vi "RT Microprocessor.vi"() -> ()   [LabVIEW 2014]
uses:
  <vilib>/FPGAPlugInAG/sbRIO-9636/niLvFpga_Open_sbRIO-9636.vi
  <vilib>/rvi/interface/common/dynamic/niFpgaDynamicAddResources.vi
  <vilib>/EmbeddedDisplay/Hitachi HD44780/Host/Public/Output (String).vi
  <vilib>/rvi/interface/nirviOpenFPGA/nirviOpenFPGA.xnode
  FPGA Bitfiles/Exercise1-OpenRu_FPGATarget_Exercise1Openand_49511F73.lvbitx
  <vilib>/EmbeddedDisplay/Hitachi HD44780/Host/HD44780 Host.lvlib
panel:
  in  "Direction":bool
  in  "Text":string="NI LabVIEW RIO Architecture"
  in  "stop":bool
  # "This VI writes the text you specify on the LCD device,\nand then shifts the text to the left or the right."
  # "Output Configuration"
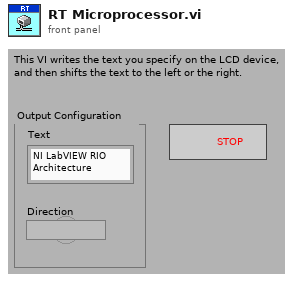
[diagram p1: front panel]
types:
  T1 = enum8{"5x8 & 2 lines", "5x10 & 1 line", "5x8 & 1 line"}
  T2 = enum8{"8x1", "8x2", "12x4", "16x1", "16x2", "16x4", "20x1", "20x2", "20x4", "24x1", "24x2", "40x2", "40x4"}
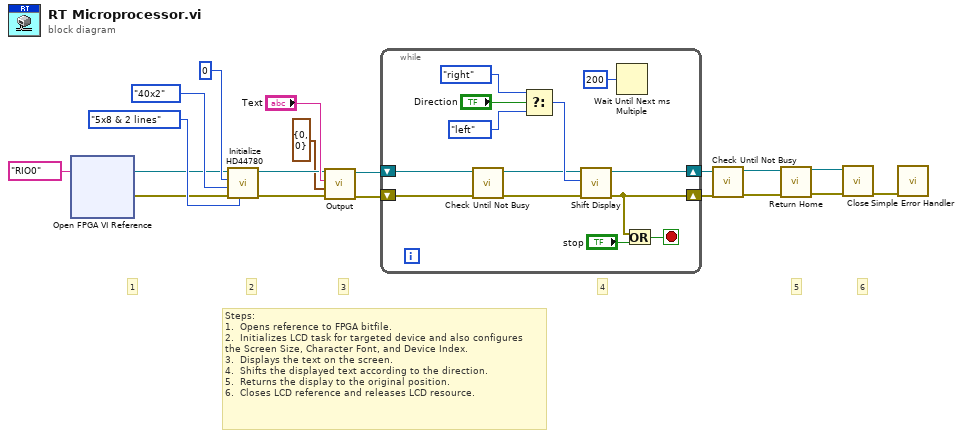
[diagram p0: block diagram]
diagram:
  # "6"
  # "5"
  # "4"
  # "3"
  # "2"
  # "1"
  # "Steps:  \n1.  Opens reference to FPGA bitfile.\n2.  Initializes LCD task for targeted device and also configures\nthe Screen Size, Character Font, and Device Index.\n3.  Displays the text on the screen.\n4.  Shifts the displayed text according to the direction.\n5.  Returns the display to the original position.\n6.  Closes LCD reference and releases LCD resource."
  n1 = xnode "Open FPGA VI Reference"("resource name"=tag "RIO0") -> ("FPGA VI Reference Out"=w3:refnum<k20>, "error out"=w2:errorcluster)  [unwired: 1 in]
  n2 = call <vilib>:"Initialize HD44780.vi"("font configuration (5x8 & 2 lines)"=T1."5x8 & 2 lines" ("font configuration"), "error in (no error)"=w2, "screen size"=T2."40x2", "device index"=i8 0, "FPGA VI Reference in"=w3) -> ("error out"=w7:errorcluster, "LCD out"=w8:refnum<class "Character LCD.lvclass">)  [unwired: 5 in]
  n3 = call-poly <vilib>:"Output.vi"("error in (no error)"=w7, "position"=cluster{"column":i8, "row":i8} {"column"=0, "row"=0}, "text"="Text", "LCD in"=w8) -> ("error out"=w4:errorcluster, "LCD out"=w5:refnum<class "Character LCD.lvclass">)  [unwired: 5 in, 1 out]
  n4 = while {
    shift-right: [w32] -> w14
    shift-left: w5 -> [w24]
    shift-right: [w21] -> w13
    shift-left: w4 -> [w23]
    stop <- w20 stop-if-true
    n5 = call "Check Until Not Busy.vi"("error in"=w23, "LCD in"=w24) -> ("error out"=w25:errorcluster, "LCD out"=w26:refnum<class "Character LCD.lvclass">)  [unwired: 8 in]
    n6 = Select(t=enum16{"left", "right"}."right" ("direction"), s="Direction", f=enum16{"left", "right"}."left" ("direction")) -> (s? t:f=w28:enum16{"left", "right"})
    n7 = call <vilib>:"Shift Display.vi"("error in (no error)"=w25, "direction"=w28, "LCD in"=w26) -> ("error out"=w21:errorcluster, "LCD out"=w32:refnum<class "Character LCD.lvclass">)  [unwired: 7 in]
    n8 = Wait Until Next ms Multiple(millisecond multiple=u32 200) -> ()  [unwired: 1 out]
    n9 = Or(x=w21, y="stop") -> (x .or. y?=w20:bool)
  }
  n10 = call "Check Until Not Busy.vi"("error in"=w13, "LCD in"=w14) -> ("error out"=w11:errorcluster, "LCD out"=w12:refnum<class "Character LCD.lvclass">)  [unwired: 8 in]
  n11 = call <vilib>:"Return Home.vi"("error in (no error)"=w11, "LCD in"=w12) -> ("error out"=w18:errorcluster, "LCD out"=w19:refnum<class "Character LCD.lvclass">)  [unwired: 8 in]
  n12 = call <vilib>:"Close.vi"("error in (no error)"=w18, "LCD in"=w19) -> ("error out"=w10:errorcluster)  [unwired: 9 in]
  n13 = call <vilib>:"Simple Error Handler.vi"("error in (no error)"=w10) -> ()  [unwired: 4 in, 5 out]
